vi "BaseTemplate_4x4x4_GOOPKernel.vi"(0 "Ref in":refnum<class "BaseTemplate_4x4x4.lvclass">, 1 "Data in":T4 {"Attribute1" format="%.2f"}, 2 "Data shared in":T2, 3 "Probe in":string, 6 "Subclass names":string[](array[string]), 7 "error in (no error)":errorcluster, 8 "Action":T3, 9 "Subclass?":bool, 10 "Object name":string, 11 "Class name":string, 13 "Misc":bool, 15 "Occurrence":refnum<k4>, 17 "Occurrence shared":refnum<k4>) -> (14 "Occurrence out":refnum<k4>, 16 "# of objects":i32, 18 "Class statistics":T1, 19 "IsSubclass?":bool, 20 "Ref out":refnum<class "BaseTemplate_4x4x4.lvclass">, 21 "Data out":T4 {"Attribute1" format="%.2f"}, 22 "Data shared out":T2, 23 "Probe out":string, 25 "Exists?":bool, 26 "Data locked?":bool, 27 "error out":errorcluster)   [LabVIEW 2012, in "BaseTemplate_4x4x4.lvclass"]
doc: "This VIs manages objects of the $CLASS$.\n\n$VERSION$"
uses:
  <resource>/Framework/Providers/Open_GDS/ClassProviders/Provider_EndevoGOOP300/Templates/BaseTemplate_4x4x4/BaseTemplate_4x4x4.lvclass
  <resource>/Framework/Providers/Open_GDS/ClassProviders/Provider_EndevoGOOP300/Templates/BaseTemplate_4x4x4/protected/ObjectAttributes.ctl
  <vilib>/addons/_goop3.llb/3GOOPStates.ctl
  <resource>/Framework/Providers/Open_GDS/ClassProviders/Provider_EndevoGOOP300/Templates/BaseTemplate_4x4x4/protected/ClassAttributes.ctl
  <vilib>/addons/_goop3.llb/3GOOPClassStatistics.ctl
  <resource>/Framework/Providers/Open_GDS/ClassProviders/Provider_EndevoGOOP300/Templates/BaseTemplate_4x4x4/BaseTemplate_4x4x4.lvclass/BaseTemplate_4x4x4.ctl
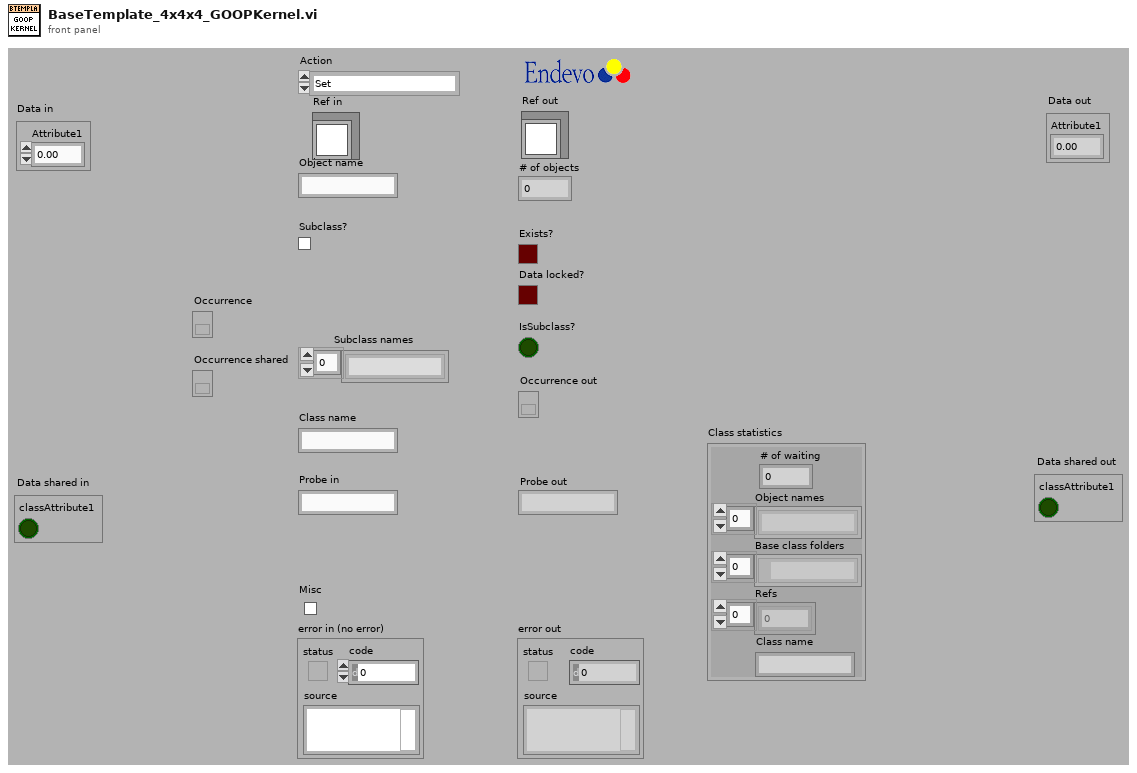
[diagram p1: front panel]
types:
  T1 = typedef "3GOOPClassStatistics.ctl" = cluster{"# of waiting":u32, "Object names":string[], "Base class folders":path[], "Refs":i32[], "Class name":string}
  T2 = typedef "BaseTemplate_4x4x4.lvclass/ClassAttributes.ctl" = cluster{"classAttribute1":bool}
  T3 = typedef "3GOOPStates.ctl" = enum16{"Set", "Get", "New", "Delete", "Clear", "Test and get", "Unlock data", "Information", "Look up existing", "New or look up existing", "Test and get shared", "Get shared", "Set shared", "Unlock shared", "Find dynamic method", "Register dynamic method", "Preload dynamic method", "Probe", "Cast to more generic", "Cast to more specific"}
  T4 = typedef "BaseTemplate_4x4x4.lvclass/ObjectAttributes.ctl" = cluster{"Attribute1":dbl}
  T5 = typedef "BaseTemplate_4x4x4.lvclass/ObjectReference.ctl" = refnum<k1>
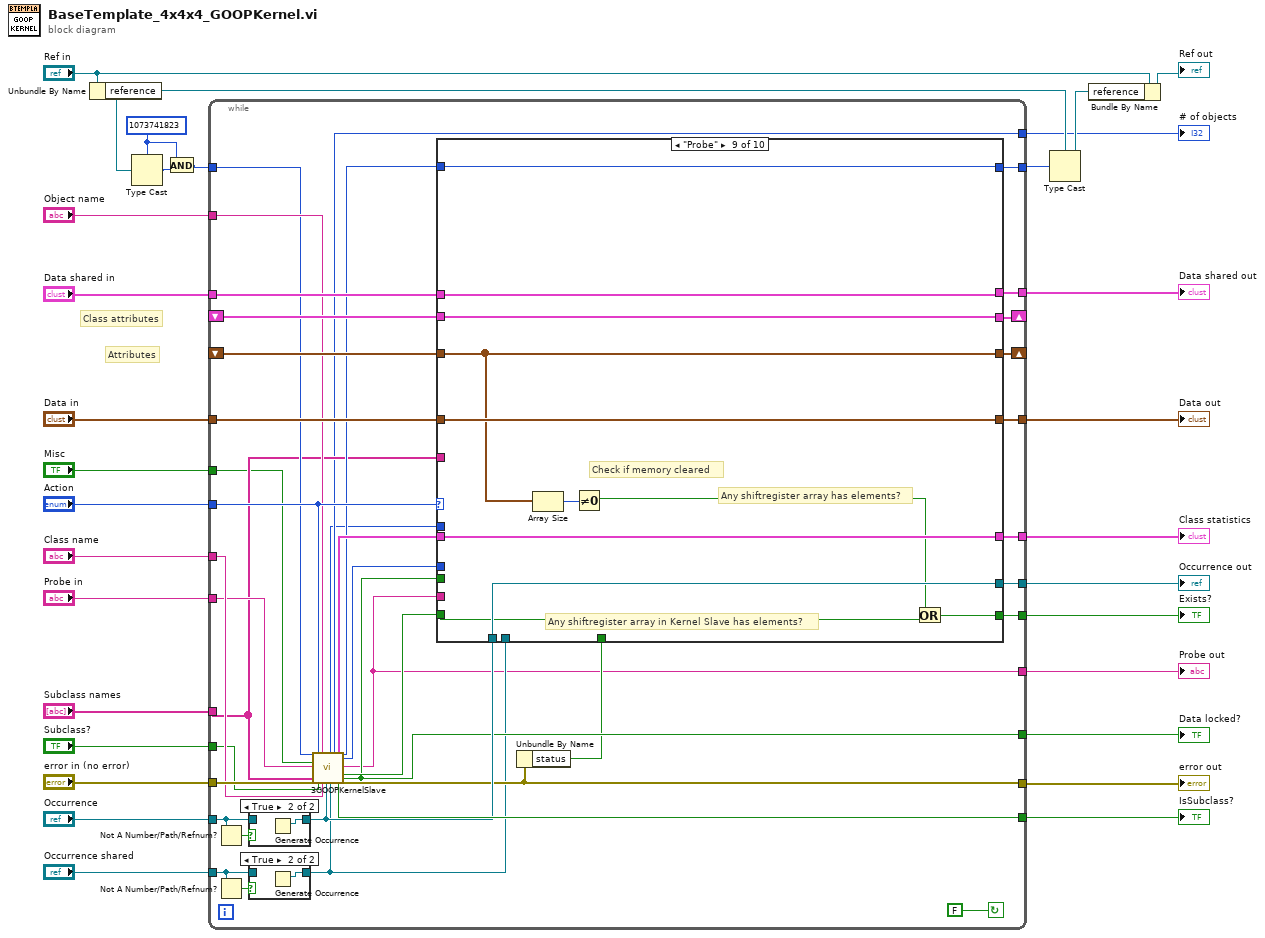
[diagram p0: block diagram]
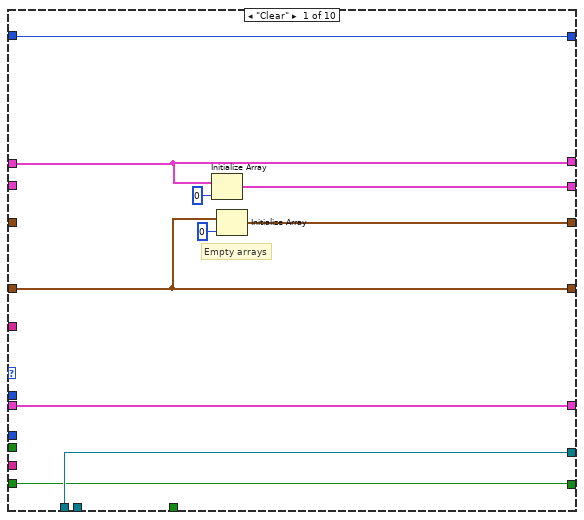
[diagram p4: hidden frame]
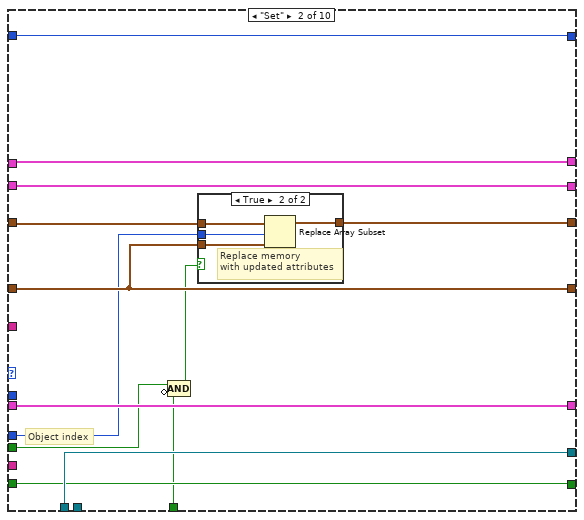
[diagram p5: hidden frame]
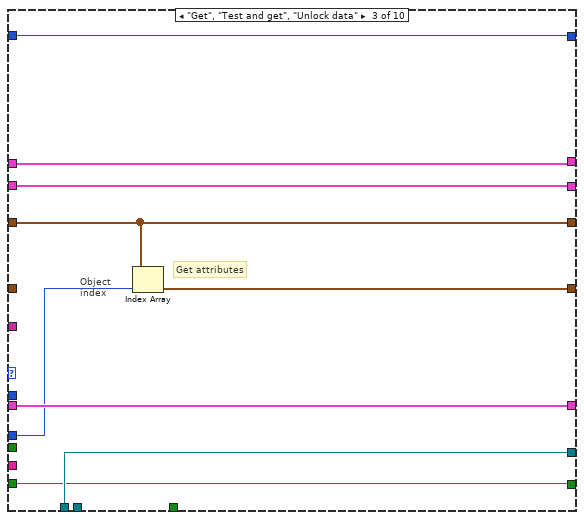
[diagram p7: hidden frame]
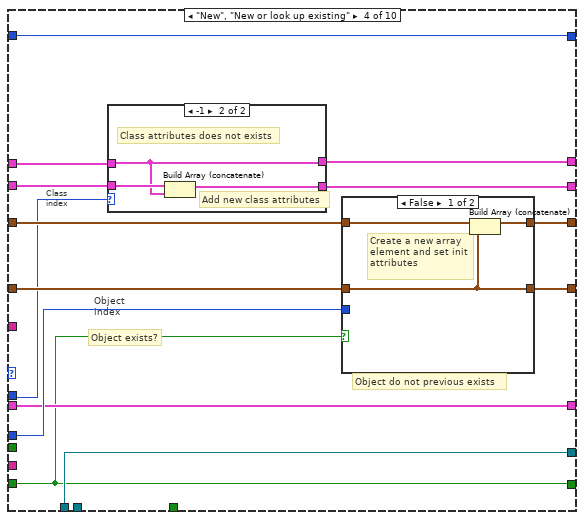
[diagram p8: hidden frame]
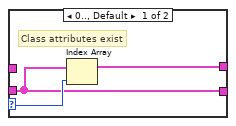
[diagram p9: hidden frame]
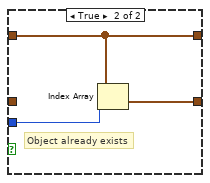
[diagram p10: hidden frame]
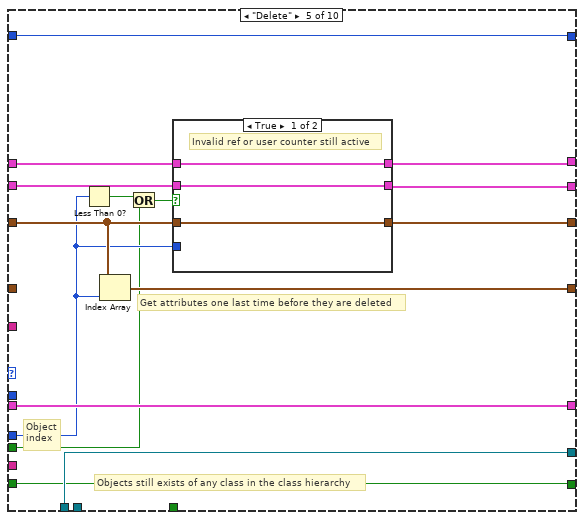
[diagram p11: hidden frame]
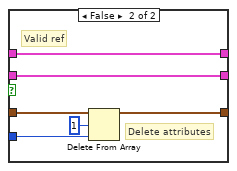
[diagram p12: hidden frame]
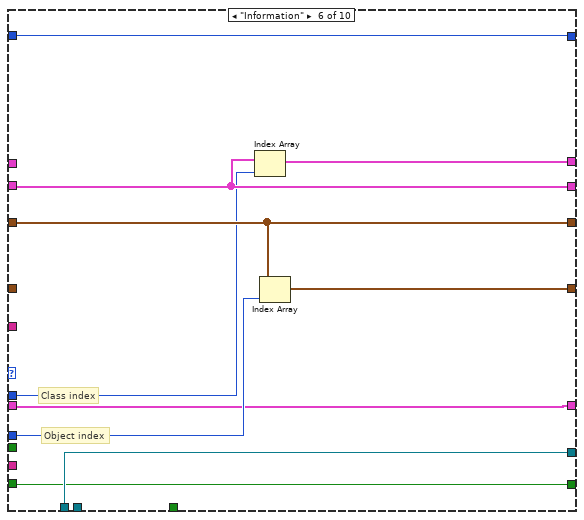
[diagram p13: hidden frame]
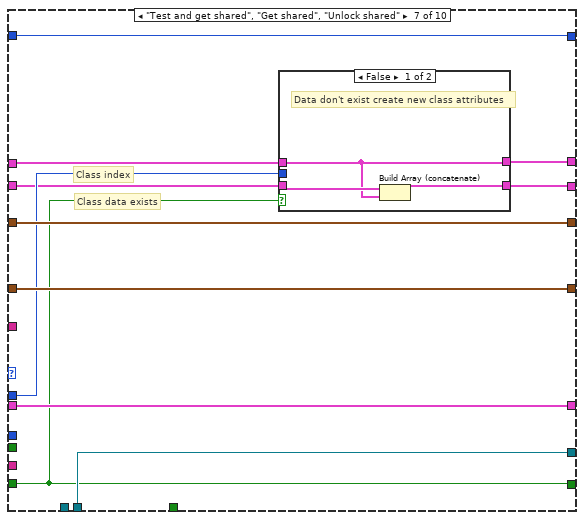
[diagram p14: hidden frame]
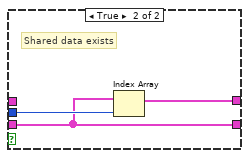
[diagram p15: hidden frame]
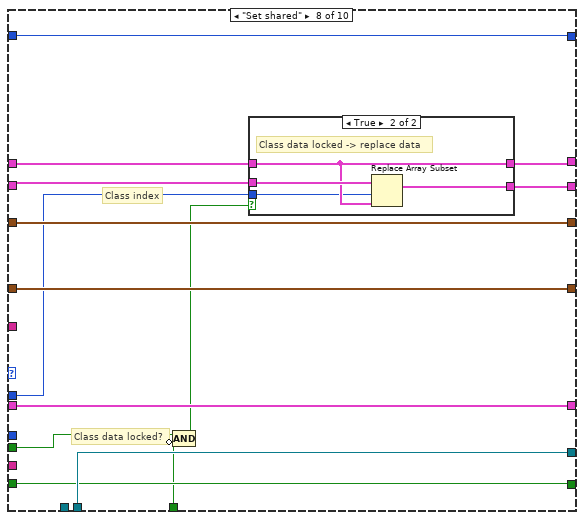
[diagram p16: hidden frame]
diagram:
  w29 = 1073741823 ("x .and. y?")
  # "Attributes"
  # "Class attributes"
  n1 = Unbundle By Name("Ref in") -> ("reference"=w26:T5)
  n2 = Type Cast(type=w29, x=w26) -> (*(type *) &x=w30:i32)
  n3 = And(x=w29, y=w30) -> (x .and. y?=w24:i32)
  n4 = while {
    tunnel: [w40] -> w5
    tunnel: [w44] -> w6
    tunnel: [w46] -> w11
    tunnel: "Misc" -> [w47]
    tunnel: [w49] -> w9
    tunnel: [w50] -> w1
    tunnel: [w61] -> w7
    tunnel: "Subclass names" -> [w48]
    tunnel: "Probe in" -> [w57]
    tunnel: [w31] -> w4
    tunnel: "Class name" -> [w59]
    tunnel: "Data shared in" -> [w62]
    shift-left: _ -> [w63]
    shift-right: [w64] -> _
    tunnel: "Object name" -> [w55]
    tunnel: [w39] -> w2
    tunnel: "error in (no error)" -> [w60]
    tunnel: "Subclass?" -> [w58]
    tunnel: [w41] -> w3
    tunnel: [w32] -> w10
    tunnel: w24 -> [w52]
    shift-left: _ -> [w67]
    shift-right: [w68] -> _
    tunnel: [w69] -> w8
    tunnel: "Action" -> [w56]
    tunnel: "Data in" -> [w66]
    tunnel: "Occurrence shared" -> [w36]
    tunnel: "Occurrence" -> [w33]
    stop <- FALSE continue-if-true
    n5 = Not A Number/Path/Refnum?(number/path/refnum=w33) -> (NaN/Path/Refnum?=w34:bool)
    n6 = Not A Number/Path/Refnum?(number/path/refnum=w36) -> (NaN/Path/Refnum?=w37:bool)
    n7 = case shown="True" w34 {
      tunnel: w33 -> [w70 _]
      tunnel: [w70 w71] -> w45
      frame False {
      }
      frame True {
        n8 = Generate Occurrence() -> (w71:refnum<k4>)
      }
    }
    n9 = case shown="True" w37 {
      tunnel: w36 -> [w72 _]
      tunnel: [w72 w73] -> w35
      frame False {
      }
      frame True {
        n10 = Generate Occurrence() -> (w73:refnum<k4>)
      }
    }
    n11 = call <vilib>:"3GOOPKernelSlave.vi"("ref in"=w52, "Misc"=w47, "Probe in"=w57, "Subclass names"=w48, "error in (no error)"=w60, "Action"=w56, "Subclass?"=w58, "Object name"=w55, "Class name"=w59, "Occurrence"=w45, "Occurrence shared"=w35) -> ("Shared index out"=w43:i32, "# of objects"=w46:i32, "Class statistics"=w53:T1, "IsSubclass?"=w50:bool, "ref out"=w51:i32, "Index out"=w54:i32, "Probe out"=w31:string, "Exists/DynamicCall?"=w42:bool, "Data locked?"=w41:bool, "error out"=w39:errorcluster)  [unwired: 6 in, 1 out]
    n12 = Unbundle By Name(w39) -> ("status"=w38:bool)
    n13 = case shown="\"Probe\"" w56 {
      tunnel: [w77 w96 w109 w121 w149 w169 w181 w200 w218 w223] -> w69
      tunnel: [w78 w94 w110 w123 w143 w170 w180 w201 w213 w224] -> w68
      tunnel: w67 -> [_ w95 w110 w124 w151 w170 w180 w201 w213 w224]
      tunnel: w66 -> [w77 w96 _ w122 _ _ w181 w200 w218 w223]
      tunnel: [w80 w93 w108 w115 w144 w166 w172 w197 w214 w225] -> w64
      tunnel: w63 -> [_ w93 w108 w117 w150 w166 w173 w198 w214 w225]
      tunnel: w62 -> [w81 w90 w105 w118 w146 _ w177 w196 w216 w226]
      tunnel: [w83 w92 w107 w119 w148 w162 w179 w199 w217 w222] -> w61
      tunnel: w41 -> [_ w86 _ _ w137 _ _ w190 _ _]
      tunnel: w54 -> [_ w91 w106 w120 w147 w168 _ _ _ _]
      tunnel: w53 -> [w83 w92 w107 w119 w148 w162 w179 w199 w217 w222]
      tunnel: w51 -> [w74 w84 w102 w111 w140 w161 w171 w188 w209 w219]
      tunnel: w42 -> [w75 w88 w103 w112 w141 w163 w174 w192 w210 w220]
      tunnel: [w81 w90 w105 w114 w145 w167 w178 w195 w216 w226] -> w49
      tunnel: w48 -> [_ _ _ _ _ _ _ _ _ _]
      tunnel: w45 -> [w76 w89 w104 w113 w142 w164 _ _ w215 w221]
      tunnel: w35 -> [_ _ _ _ _ _ w175 w193 _ _]
      tunnel: [w76 w89 w104 w113 w142 w164 w175 w193 w215 w221] -> w44
      tunnel: w43 -> [_ _ _ w116 _ w165 w176 w194 _ _]
      tunnel: [w75 w88 w103 w112 w141 w163 w174 w192 w211 w220] -> w40
      tunnel: w38 -> [_ w87 _ _ _ _ _ w191 _ _]
      tunnel: [w74 w84 w102 w111 w140 w161 w171 w188 w209 w219] -> w32
      tunnel: w31 -> [_ _ _ _ _ _ _ _ _ _]
      frame "Clear" {
        # "Empty arrays"
        n14 = Initialize Array(w81, 0 ("Dimension Size")) -> (w80:T2[])
        n15 = Initialize Array(w77, 0 ("Dimension Size")) -> (w78:T4[])
      }
      frame "Set" {
        # "Object index"
        n16 = Compound Arithmetic op=AND(w86, invert w87) -> (w85:bool)
        n17 = case shown="True" w85 {
          tunnel: w96 -> [_ w101]
          tunnel: w95 -> [w97 w100]
          tunnel: [w97 w99] -> w94
          tunnel: w91 -> [_ w98]
          frame False {
            # "Attributes not locked!"
          }
          frame True {
            # "Replace memory\nwith updated attributes"
            n18 = Replace Array Subset(array=w100, new element=w101, index=w98) -> (w99:T4[])
          }
        }
      }
      frame "Get", "Test and get", "Unlock data" {
        # "Object\nindex"
        # "Get attributes"
        n19 = Index Array(array=w110, index=w106) -> (element=w109:T4)
      }
      frame "New", "New or look up existing" {
        # "Object exists?"
        # "Object\nindex"
        # "Class\nindex"
        n20 = case shown="-1" w116 {
          selector: w116 -> [w127 _]
          tunnel: w118 -> [_ w128]
          tunnel: w117 -> [w126 w130]
          tunnel: [w126 w129] -> w115
          tunnel: [w125 w128] -> w114
          frame 0.., Default {
            # "Class attributes exist"
            n21 = Index Array(array=w126, index=w127) -> (element=w125:T2)
          }
          frame -1 {
            # "Add new class attributes"
            # "Class attributes does not exists"
            n22 = Build Array (concatenate)(w130, w128) -> (w129:T2[])
          }
        }
        n23 = case shown="False" w112 {
          tunnel: w124 -> [w133 w136]
          tunnel: [w132 w136] -> w123
          tunnel: w122 -> [w131 _]
          tunnel: [w131 w135] -> w121
          tunnel: w120 -> [_ w134]
          frame False {
            # "Object do not previous exists"
            # "Create a new array \nelement and set init\nattributes"
            n24 = Build Array (concatenate)(w133, w131) -> (w132:T4[])
          }
          frame True {
            # "Object already exists"
            n25 = Index Array(array=w136, index=w134) -> (element=w135:T4)
          }
        }
      }
      frame "Delete" {
        # "Objects still exists of any class in the class hierarchy"
        # "Object\nindex"
        # "Get attributes one last time before they are deleted"
        n26 = Less Than 0?(x=w147) -> (x < 0?=w138:bool)
        n27 = Index Array(array=w151, index=w147) -> (element=w149:T4)
        n28 = Or(x=w138, y=w137) -> (x .or. y?=w139:bool)
        n29 = case shown="True" w139 {
          tunnel: w151 -> [w154 w159]
          tunnel: [w154 w158] -> w143
          tunnel: w147 -> [_ w156]
          tunnel: w150 -> [w153 w157]
          tunnel: [w153 w157] -> w144
          tunnel: w146 -> [w152 w155]
          tunnel: [w152 w155] -> w145
          frame True {
            # "Invalid ref or user counter still active"
          }
          frame False {
            # "Delete attributes"
            # "Valid ref"
            n30 = Delete From Array(array=w159, length=1 ("Length"), index=w156) -> (array with subset deleted=w158:T4[])  [unwired: 1 out]
          }
        }
      }
      frame "Information" {
        # "Object index"
        # "Class index"
        n31 = Index Array(array=w166, index=w165) -> (element=w167:T2)
        n32 = Index Array(array=w170, index=w168) -> (element=w169:T4)
      }
      frame "Test and get shared", "Get shared", "Unlock shared" {
        # "Class index"
        # "Class data exists"
        n33 = case shown="False" w174 {
          tunnel: [w182 w186] -> w178
          tunnel: w173 -> [w184 w185]
          tunnel: w176 -> [_ w187]
          tunnel: w177 -> [w182 _]
          tunnel: [w183 w185] -> w172
          frame False {
            # "Data don't exist create new class attributes"
            n34 = Build Array (concatenate)(w184, w182) -> (w183:T2[])
          }
          frame True {
            # "Shared data exists"
            n35 = Index Array(array=w185, index=w187) -> (element=w186:T2)
          }
        }
      }
      frame "Set shared" {
        # "Class data locked?"
        # "Class index"
        n36 = Compound Arithmetic op=AND(w190, invert w191) -> (w189:bool)
        n37 = case shown="True" w189 {
          tunnel: w198 -> [w203 w207]
          tunnel: [w203 w206] -> w197
          tunnel: w196 -> [w202 w205]
          tunnel: [w202 w205] -> w195
          tunnel: w194 -> [_ w204]
          frame False {
            # "Shared data not locked -> error do not update"
          }
          frame True {
            # "Class data locked -> replace data"
            n38 = Replace Array Subset(array=w207, new element=w205, index=w204) -> (w206:T2[])
          }
        }
      }
      frame "Probe" {
        # "Any shiftregister array in Kernel Slave has elements?"
        # "Any shiftregister array has elements?"
        # "Check if memory cleared"
        n39 = Array Size(array=w213) -> (size(s)=w212:i32)
        n40 = Not Equal To 0?(x=w212) -> (x != 0?=w208:bool)
        n41 = Or(x=w208, y=w210) -> (x .or. y?=w211:bool)
      }
      frame "Look up existing", "Cast to more generic", "Cast to more specific", Default {
      }
    }
  }
  "Data out" <- w8
  "Data locked?" <- w3
  "error out" <- w2
  "Exists?" <- w5
  "Data shared out" <- w9
  "Probe out" <- w4
  "Class statistics" <- w7
  "IsSubclass?" <- w1
  "# of objects" <- w11
  "Occurrence out" <- w6
  n42 = Type Cast(type=w26, x=w10) -> (*(type *) &x=w25:T5)
  n43 = Bundle By Name(cluster="Ref in", "reference"=w25) -> (→"Ref out":refnum<class "BaseTemplate_4x4x4.lvclass">)
